vi "UDP Data Link - Driver Utilities - RT FIFO Read.vi"(5 "SeqNum FIFO Index":i32, 6 "poll rate in us":u32, 7 "Current SeqNum":dbl, 8 "error in (no error)":errorcluster, 9 "timeout in us":u32, 10 "element":dbl[](array[numeric]), 11 "rt fifo (dbl array)":refnum<k33>) -> (0 "error out":errorcluster, 1 "empty?":bool, 2 "element out":dbl[](array[numeric]), 3 "rt fifo out (dbl array)":refnum<k33>, 4 "# elements":u32)   [LabVIEW 2015, in "UDP Data Link Engine.lvlib"]
doc: "This VI implements an RT FIFO Read with timeout resolution in the microsecond. RT FIFO Read's normally only have msec timeouts. This VI also specifies a polling rate that is also specified in microseconds. It will poll the RT FIFO at the rate requested by the polling rate. In between polls, this VI puts its thread to sleep. When awoken, this VI checks if it has exceeded the timeout. If there is a mismatch between the poll rate and the timeout values, it's possible for this VI to execute longer than the time specified in timeout. It will return when either reading a new element from the FIFO or exceeding the timeout value when checked.\n\nNote that this VI also avoids a bug that destroys the RT FIFO reference when requesting a read from FIFO with timeout if the FIFO is set to perform a blocking read inside of a Time-Critical Priority VI."
uses:
  UDP Data Link Engine.lvlib
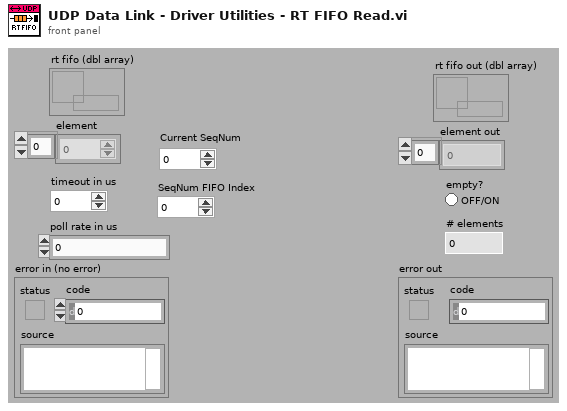
[diagram p1: front panel]
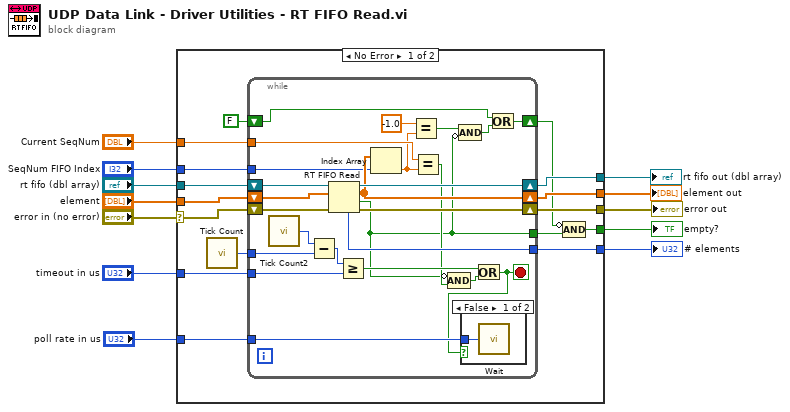
[diagram p0: block diagram]
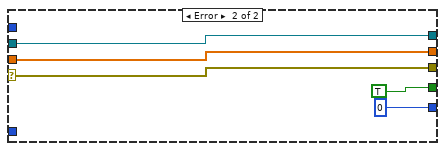
[diagram p3: hidden frame]
diagram:
  n1 = case shown="No Error" "error in (no error)" {
    selector: "error in (no error)" -> [w19 w59]
    tunnel: "timeout in us" -> [w27 _]
    tunnel: [w14 TRUE ("empty?")] -> w11
    tunnel: "rt fifo (dbl array)" -> [w25 w57]
    tunnel: [w24 w57] -> w9
    tunnel: [w23 w58] -> w8
    tunnel: "element" -> [w22 w58]
    tunnel: [w21 w59] -> w6
    tunnel: [w20 u32 0 ("# elements")] -> w5
    tunnel: "poll rate in us" -> [w18 _]
    tunnel: "SeqNum FIFO Index" -> [w17 _]
    tunnel: "Current SeqNum" -> [w16 _]
    frame No Error {
      n2 = call "Tick Count"() -> ("Tick Count(uSec)"=w28:u32)
      n3 = while {
        tunnel: w28 -> [w52]
        tunnel: w27 -> [w50]
        tunnel: [w29] -> w26
        shift-right: [w47] -> w24
        shift-left: w25 -> [w48]
        shift-right: [w40] -> w23
        shift-left: w22 -> [w46]
        shift-right: [w44] -> w21
        shift-left: w19 -> [w45]
        tunnel: [w43] -> w20
        tunnel: w18 -> [w42]
        tunnel: w17 -> [w39]
        tunnel: w16 -> [w38]
        shift-right: [w31] -> w13
        shift-left: FALSE -> [w30]
        stop <- w36 stop-if-true
        n4 = call "Tick Count2"() -> ("Tick Count(uSec)"=w53:u32)
        n5 = Subtract(x=w53, y=w52) -> (x-y=w51:u32)
        n6 = RT FIFO Read(0:w48, 1:w46, 3:w45) -> (7:w43:u32, 8:w47:refnum<k33>, 9:w40:dbl[], 10:w29:bool, 11:w44:errorcluster)  [unwired: 1 in]
        n7 = Greater Or Equal?(x=w51, y=w50) -> (x >= y?=w49:bool)
        n8 = Index Array(array=w40, index=w39) -> (element=w35:dbl)
        n9 = Equal?(x=-1.0, y=w35) -> (x = y?=w33:bool)
        n10 = Equal?(x=w38, y=w35) -> (x = y?=w37:bool)
        n11 = Compound Arithmetic op=AND(invert w29, w37) -> (w41:bool)
        n12 = Compound Arithmetic op=AND(w33, invert w29) -> (w32:bool)
        n13 = Or(x=w49, y=w41) -> (x .or. y?=w36:bool)
        n14 = case shown="False" w36 {
          tunnel: w42 -> [w54 _]
          frame False {
            n15 = call "Wait"("Count(uSec)"=w54) -> ()  [unwired: 1 out]
          }
          frame True {
          }
        }
        n16 = Or(x=w30, y=w32) -> (x .or. y?=w31:bool)
      }
      n17 = Compound Arithmetic op=AND(invert w13, w26) -> (w14:bool)
    }
    frame Error {
    }
  }
  "empty?" <- w11
  "rt fifo out (dbl array)" <- w9
  "element out" <- w8
  "error out" <- w6
  "# elements" <- w5
